vi "TEST - Cluster to Array of VData.vi"(8 "error in (no error)":errorcluster) -> (0 "error out":errorcluster, 2 "pass":bool)   [LabVIEW 2020, in "test_openg_array.lvlib"]
uses:
  test_openg_array.lvlib
  <userlib>/_OpenG.lib/error/error.llb/openg_error.lvlib
  source/library/openg_variant.lvlib
  <vilib>/addons/_JKI Toolkits/Caraya/classes/Test/Test.lvclass
  <vilib>/addons/_JKI Toolkits/Caraya/classes/Assert/Assert.lvclass
  <vilib>/addons/_JKI Toolkits/Caraya/classes/Assert/Assert True.vi
panel:
  out "expected result":errorcluster
  out "result":errorcluster
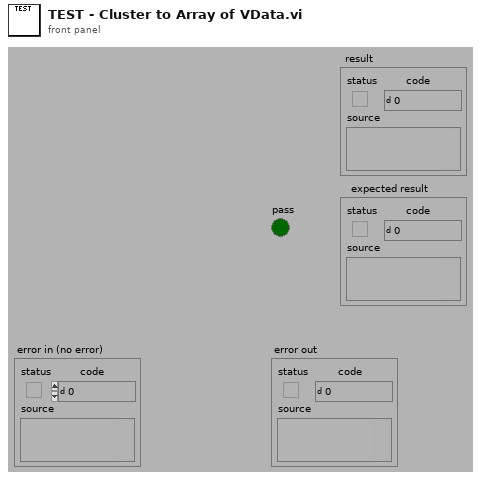
[diagram p1: front panel]
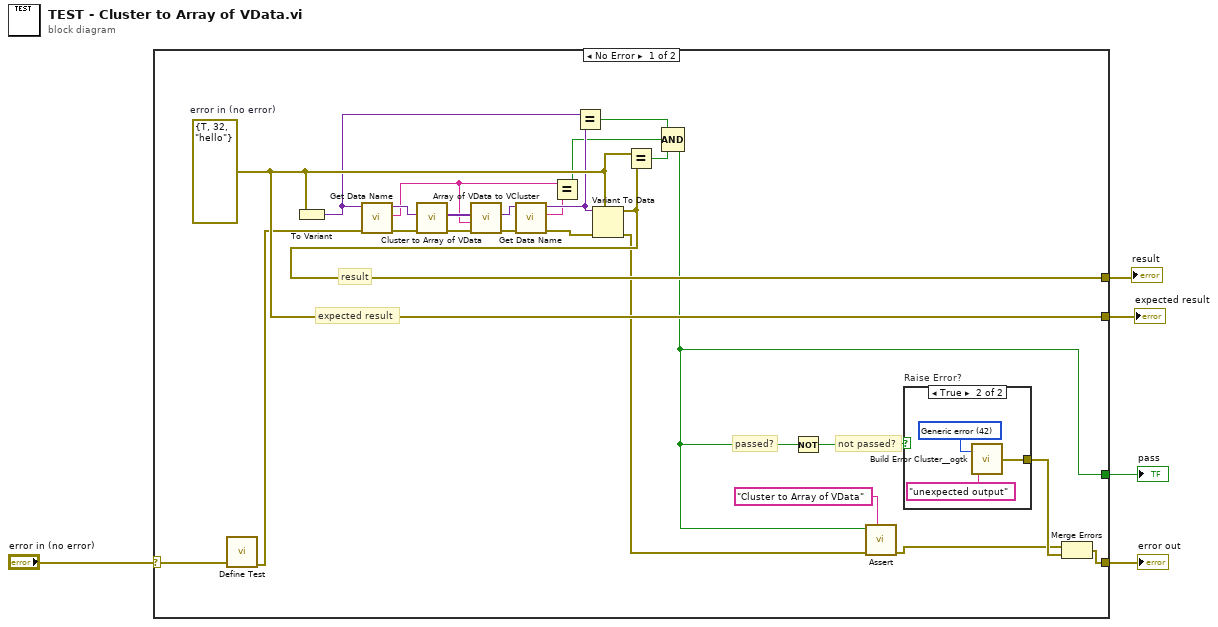
[diagram p0: block diagram]
diagram:
  n1 = case shown="No Error" "error in (no error)" {
    selector: "error in (no error)" -> [w10 w34]
    tunnel: [w8 _] -> w5
    tunnel: [w30 w34] -> w3
    tunnel: [w22 _] -> w2
    tunnel: [w23 _] -> w1
    frame No Error {
      w23 = errorcluster {"status"=TRUE, "code"=32, "source"="hello"}  # error in (no error)
      # "result"
      # "expected result"
      # "not passed?"
      # "passed?"
      n2 = call <vilib>:"Define Test.vi"("error in (no error)"=w10) -> ("error out"=w9:errorcluster)  [unwired: 9 in, 1 out]
      n3 = To Variant(anything=w23) -> (Variant=w21:variant)
      n4 = call "Get Data Name.vi"("error in (no error)"=w9, "Data"=w21) -> ("error out"=w19:errorcluster, "Data Name"=w13:string, "Data dup"=w20:variant)  [unwired: 7 in]
      n5 = call "Cluster to Array of VData.vi"("error in (no error)"=w19, "Cluster"=w20) -> ("error out"=w26:errorcluster, "Array of VData"=w27:variant[])  [unwired: 8 in]
      n6 = call "Array of VData to VCluster.vi"("error in (no error)"=w26, "Cluster Name"=w13, "Array"=w27) -> ("error out"=w18:errorcluster, "VCluster"=w17:variant)  [unwired: 7 in]
      n7 = call "Get Data Name.vi"("error in (no error)"=w18, "Data"=w17) -> ("error out"=w15:errorcluster, "Data Name"=w14:string, "Data dup"=w16:variant)  [unwired: 7 in]
      n8 = Equal?(x=w13, y=w14) -> (x = y?=w12:bool)
      n9 = Equal?(x=w21, y=w16) -> (x = y?=w24:bool)
      n10 = Variant To Data(error in=w15, type=w23, Variant=w16) -> (data=w22:errorcluster, error out=w6:errorcluster)
      n11 = Equal?(x=w23, y=w22) -> (x = y?=w25:bool)
      n12 = Compound Arithmetic op=AND(w24, w12, w25) -> (w8:bool)
      n13 = Not(x=w8) -> (.not. x?=w28:bool)
      n14 = call-poly <vilib>:"Assert.vi"("Label"="Cluster to Array of VData" ("Label (VI Title)"), "error in (no error)"=w6, "True?"=w8) -> ("error out"=w7:errorcluster)  [unwired: 7 in, 1 out]
      n15 = case "Raise Error?" shown="True" w28 {
        tunnel: [_ w31] -> w29
        frame False {
        }
        frame True {
          w32 = 42 items=["No error", "Argument error", "Memory is full", "Out of zone", "End of file", "File already open", "Generic file I/O error", "File not found", "File permission error", "Disk is full", "Duplicate path", "Too many files open", "System feature not enabled", "Resource file not found", "Cannot add resource", "Resource not found", "Image not found", "Image memory error", "Pen does not exist", "Config type invalid", "Config token not found", "Config parse error", "Config memory error", "Bad external code format", "Bad external code offset", "External code not present", "Null window", "Destroy window error", "Null menu", "Print aborted", "Bad print record", "Print driver error", "Windows error during printing", "Memory error during printing", "Print dialog error", "Generic print error", "Invalid device refnum", "Device not found", "Device parameter error", "Device unit error", "Cannot open device", "Device call aborted", "Generic error", "Cancelled by user", "Object ID too low", "Object ID too high", "Object not in heap", "Unknown heap", "Unknown object (invalid DefProc)", "Unknown object (DefProc not in table)", "Message out of range", "Invalid (null) method", "Unknown message", "Manager call not supported", "Bad address", "Network operation in progress", "Network operation timed out", "Connection is busy", "Network attribute not supported", "Network error", "Address in use", "System out of memory", "Connection aborted", "Connection refused", "Not connected", "Already connected", "Connection closed", "Initialization error (interapplication manager)", "Bad occurrence", "Wait on unbound occurrence handler", "Occurrence queue overflow", "Datalog type conflict", "Unused", "Unrecognized type (interapplication manager)", "Memory corrupt", "Failed to make temporary DLL", "Old CIN version", "Drag socket not found", "Failed to load drop-object", "Failed to register OLE object", "Failed to release OLE object", "Format specifier type mismatch", "Unknown format specifier", "Too few format specifiers", "Too many format specifiers", "Scan failed", "Newer CIN version", "Error converting to variant", "Runtime menu error", "Password tampered", "Variant attribute not found", "Incompatible variant data type", "Event data is not available", "Event Store is not present", "Occurrence is not found", "Event Queue is not created", "Event info is not available", "Refnum passed is NULL", "Error retrieving Class GUID", "Error retrieving CoClass GUID", "Error retrieving TypeLib GUID.", "Bad built application magic bytes.", "Specific driver is different from the specific driver associated with the Logical Name.", "There is no session opened to the class driver.", "Max Error", "MAX - Error with config objects", "MAX - Error loading configuration", "MAX - Group not supported"]
          n16 = call <userlib>:"Build Error Cluster__ogtk.vi"("String to Prepend to source (\"\")"="unexpected output" ("String to Prepend to source (\"\")"), "code"=w32) -> ("error out"=w31:errorcluster)
        }
      }
      n17 = Merge Errors(w7, w29) -> (w30:errorcluster)
    }
    frame Error {
    }
  }
  "pass" <- w5
  "error out" <- w3
  "result" <- w2
  "expected result" <- w1
